vi "readDataFromJobsListFiles.vi"(8 "errorIn":errorcluster) -> (0 "errorOut":errorcluster, 3 "staitisticsData":T1)   [LabVIEW 2025]
uses:
  control/statisticsData.ctl
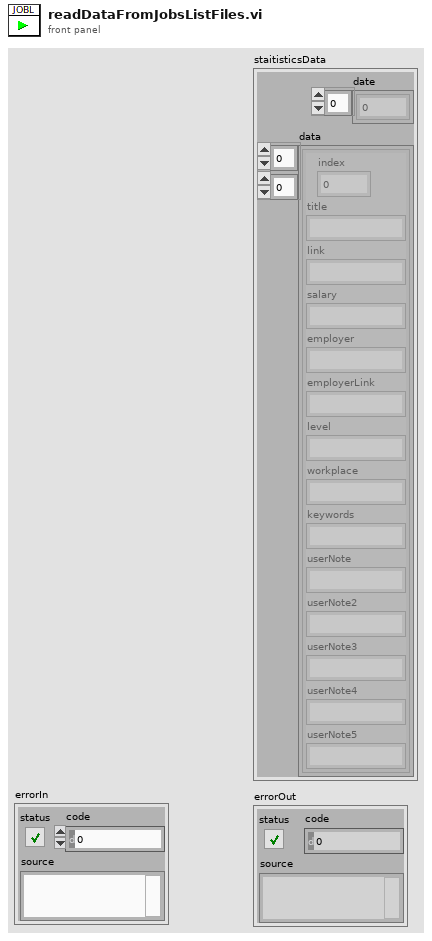
[diagram p1: front panel]
types:
  T1 = typedef "statisticsData.ctl" = cluster{"date":dbl[], "data":cluster{"index":i32, "title":string, "link":string, "salary":string, "employer":string, "employerLink":string, "level":string, "workplace":string, "keywords":string, "userNote":string, "userNote2":string, "userNote3":string, "userNote4":string, "userNote5":string}[][]}
  T2 = cluster{"index":i32, "title":string, "link":string, "salary":string, "employer":string, "employerLink":string, "level":string, "workplace":string, "keywords":string, "userNote":string, "userNote2":string, "userNote3":string, "userNote4":string, "userNote5":string}[]
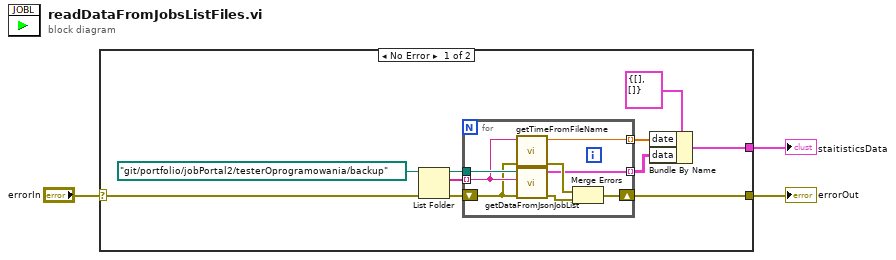
[diagram p0: block diagram]
diagram:
  n1 = case shown="No Error" "errorIn" {
    selector: "errorIn" -> [w4 w22]
    tunnel: [w13 w22] -> w3
    tunnel: [w12 _] -> w2
    frame No Error {
      n2 = List Folder(path=path "/git/portfolio/jobPortal2/testerOprogramowania/backup", error in=w4) -> (path out=w10:path, filenames=w11:string[], error out=w9:errorcluster)  [unwired: 2 in, 1 out]
      n3 = for {
        tunnel: w11 -> [w20] mode=indexing
        tunnel: w10 -> [w21]
        shift-right: [w16] -> w13
        shift-left: w9 -> [w19]
        tunnel: [w15] -> w5 mode=indexing
        tunnel: [w14] -> w6 mode=indexing
        n4 = call "getTimeFromFileName.vi"("errorIn"=w19, "fileName"=w20) -> ("errorOut"=w18:errorcluster, "date"=w14:dbl)  [unwired: 8 in]
        n5 = call "getDataFromJsonJobList.vi"("errorIn"=w19, "jobFileName"=w20, "jobFilesFolderPath"=w21) -> ("errorOut"=w17:errorcluster, "data"=w15:T2)  [unwired: 7 in]
        n6 = Merge Errors(w18, w17) -> (w16:errorcluster)
      }
      n7 = Bundle By Name(cluster=T1 {"date"=[], "data"=[]} ("staisticsData"), "date"=w6, "data"=w5) -> (w12:T1)
    }
    frame Error {
    }
  }
  "errorOut" <- w3
  "staitisticsData" <- w2
